vi "UpdateProject.vi"(8 "error in (no error)":errorcluster, 10 "Version":u32=2021, 11 "Project Path":path=path "\\\\vmware-host\\Shared Folders/_Repo/NI-XNET-Monitor-Custom-Device/Source/NI-XNET Monitor Custom Device.lvproj") -> (0 "error out":errorcluster, 3 "Project Path Out":path=path "\\\\vmware-host\\Shared Folders/_Repo/NI-XNET-Monitor-Custom-Device/Source/NI-XNET Monitor Custom Device.lvproj")   [LabVIEW 2020, in "Library Builder.lvclass"]
uses:
  Library Builder.lvclass
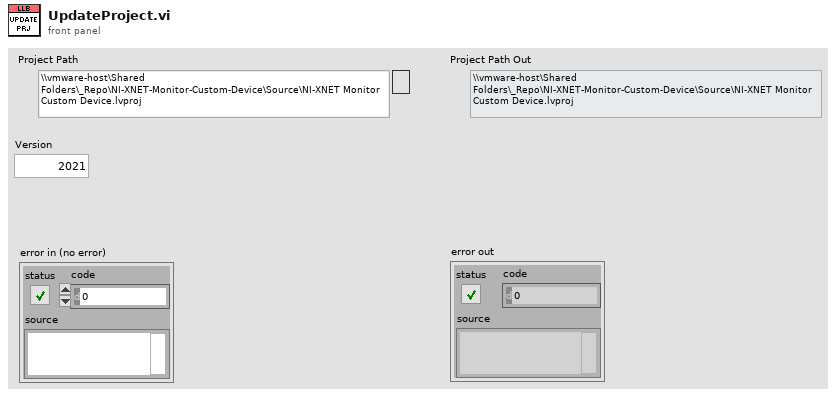
[diagram p1: front panel]
types:
  T1 = enum16{"open", "replace", "create", "open or create", "replace or create", "replace or create with confirmation"}
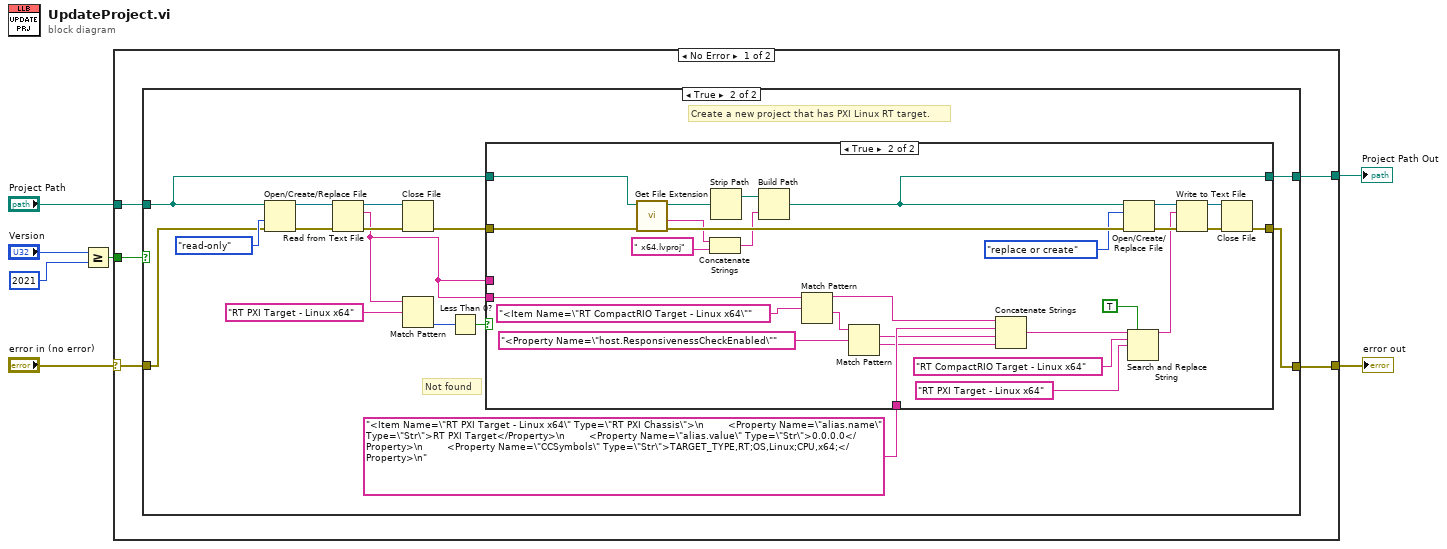
[diagram p0: block diagram]
diagram:
  n1 = Greater Or Equal?(x="Version", y=u32 2021 ("Version")) -> (x >= y?=w2:bool)
  n2 = case shown="No Error" "error in (no error)" {
    selector: "error in (no error)" -> [w10 w60]
    tunnel: "Project Path" -> [w12 _]
    tunnel: [w11 w60] -> w4
    tunnel: w2 -> [w9 _]
    tunnel: [w8 _] -> w1
    frame No Error {
      n3 = case shown="True" w9 {
        tunnel: w12 -> [w13 w20]
        tunnel: [w14 w19] -> w11
        tunnel: w10 -> [w14 w24]
        tunnel: [w13 w15] -> w8
        frame False {
        }
        frame True {
          # "Create a new project that has PXI Linux RT target."
          # "Not found"
          n4 = Open/Create/Replace File(file path (use dialog)=w20, error in=w24, access (0:read/write)=enum16{"read/write", "read-only", "write-only"}."read-only") -> (refnum out=w27:refnum<file>, error out=w29:errorcluster)  [unwired: 3 in, 1 out]
          n5 = Read from Text File(file (use dialog)=w27, error in=w29) -> (refnum out=w26:refnum<file>, text=w16:string, error out=w28:errorcluster)  [unwired: 2 in, 1 out]
          n6 = Close File(refnum=w26, error in=w28) -> (error out=w21:errorcluster)  [unwired: 1 out]
          n7 = Match Pattern(string=w16, regular expression="RT PXI Target - Linux x64") -> (offset past match=w22:i32)  [unwired: 1 in, 3 out]
          n8 = Less Than 0?(x=w22) -> (x < 0?=w18:bool)
          n9 = case shown="True" w18 {
            tunnel: w21 -> [w31 w57]
            tunnel: w20 -> [w30 w59]
            tunnel: [w31 w58] -> w19
            tunnel: "<Item Name=\"RT PXI Target - Linux x64\" Type=\"RT PXI Chassis\">\n        <Property Name=\"alias.name\" Type=\"Str\">RT PXI Target</Property>\n        <Property Name=\"alias.value\" Type=\"Str\">0.0.0.0</Property>\n        <Property Name=\"CCSymbols\" Type=\"Str\">TARGET_TYPE,RT;OS,Linux;CPU,x64;</Property>\n" -> [_ w55]
            tunnel: w16 -> [_ _]
            tunnel: w16 -> [_ w53]
            tunnel: [w30 w41] -> w15
            frame False {
            }
            frame True {
              n10 = call <vilib>:"Get File Extension.vi"("error in (no error)"=w57, "file"=w59) -> ("error out"=w48:errorcluster, "filename without extension"=w44:string, "dup file"=w47:path)  [unwired: 5 in, 2 out]
              n11 = Concatenate Strings(w44, " x64.lvproj" ("string")) -> (w43:string)
              n12 = Strip Path(path=w47) -> (stripped path=w46:path)  [unwired: 1 out]
              n13 = Build Path(base path=w46, name or relative path=w43) -> (appended path=w41:path)
              n14 = Match Pattern(string=w53, regular expression="<Item Name=\"RT CompactRIO Target - Linux x64\"") -> (before substring=w56:string, after substring=w40:string)  [unwired: 1 in, 2 out]
              n15 = Match Pattern(string=w40, regular expression="<Property Name=\"host.ResponsivenessCheckEnabled\"") -> (match substring=w33:string, after substring=w32:string)  [unwired: 1 in, 2 out]
              n16 = Concatenate Strings(w56, w55, w33, w32) -> (w38:string)
              n17 = Open/Create/Replace File(file path (use dialog)=w41, error in=w48, operation (0:open)=T1."replace or create") -> (refnum out=w51:refnum<file>, error out=w50:errorcluster)  [unwired: 3 in, 1 out]
              n18 = Search and Replace String(replace all?=TRUE ("replace all? (F)"), input string=w38, search string="RT CompactRIO Target - Linux x64", replace string="RT PXI Target - Linux x64") -> (result string=w35:string)  [unwired: 4 in, 3 out]
              n19 = Write to Text File(file (use dialog)=w51, text=w35, error in=w50) -> (refnum out=w52:refnum<file>, error out=w49:errorcluster)  [unwired: 1 in, 1 out]
              n20 = Close File(refnum=w52, error in=w49) -> (error out=w58:errorcluster)  [unwired: 1 out]
            }
          }
        }
      }
    }
    frame Error {
    }
  }
  "error out" <- w4
  "Project Path Out" <- w1
